vi "Offset_and_Ampltiude_subvi.vi"(1 "Offset":dbl, 2 "Amplitude":dbl(knob) scale=0.0..1000.0, 3 "Y":dbl[](array[numeric])) -> (0 "Array":dbl[](array[numeric]))   [LabVIEW 2020]
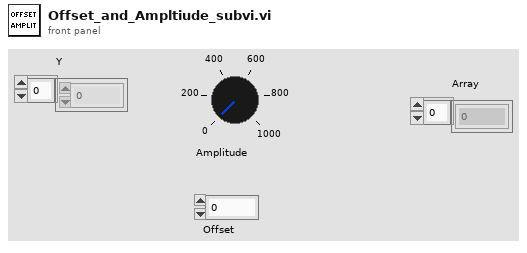
[diagram p1: front panel]
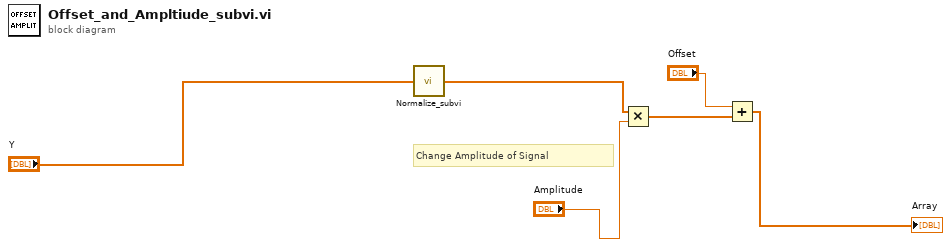
[diagram p0: block diagram]
diagram:
  # "Change Amplitude of Signal"
  n1 = call "Normalize_subvi.vi"("Y"="Y") -> ("Array"=w1:dbl[])
  n2 = Multiply(x=w1, y="Amplitude") -> (x*y=w2:dbl[])
  n3 = Add(x="Offset", y=w2) -> (x+y=→"Array":dbl[])
